vi "slide.vi"() -> ()   [LabVIEW 2023]
panel:
  in  "Tab Control":enum32{"Num Ctris", "Num Ctris i32"}(tab)
  in  "Knob":dbl(knob) scale=0.0..10.0
  in  "Dial":dbl(knob) scale=0.0..10.0
  in  "Vertical full Slide":dbl(slide) scale=0.0..10.0
  in  "Vertical Pointer Slide":dbl(slide) scale=0.0..10.0
  in  "Color Box":u32(colorbox)
  in  "Side Pointer Slide":dbl(slide) scale=0.0..10.0
  in  "Side Full Slide":dbl(slide) scale=0.0..10.0
  in  "Num Ctrl":dbl
  out "Numeric":dbl
  out "Side Full":dbl
  out "Side Pointer":dbl
  out "Vertical Full":dbl
  out "Vertical Pointer":dbl
  out "Knob_Value":dbl
  out "Dial Value":dbl
  out "Color DEC":u32
  out "Color BIN":u32 format="%b"
  out "Color OCT":u32 format="%o"
  out "Color HEX":u32 format="%x"
  in  "Knob 2":i32(knob) scale=0.0..10.0
  in  "Dial 2":i32(knob) scale=0.0..10.0
  in  "Vertical full Slide 2":i32(slide) scale=0.0..10.0
  in  "Vertical Pointer Slide  2":i32(slide) scale=0.0..10.0
  in  "Color Box 2":u32(colorbox)
  in  "Side Pointer Slide  2":i32(slide) scale=0.0..10.0
  in  "Side Full Slide  2":i32(slide) scale=0.0..10.0
  in  "Num Ctrl 2":i32
  out "Numeric 2":i32
  out "Side Full 2":i32
  out "Side Pointer 2":i32
  out "Vertical Full 2":i32
  out "Vertical Pointer 2":i32
  out "Knob_Value 2":i32
  out "Dial Value 2":i32
  out "u32 DEC":u32
  out "u32 HEX":u32 format="%x"
  out "u32 OCT":u32 format="%o"
  out "u32 BIN":u32 format="%b"
  in  "stop":bool
  # "Express内のNum  Ctrlsのアイコンの動きを知るためのVIです。\nDBL（少数を含む）とi32（整数）２種類の型で動きが確認できます。\nプログラム終了したい場合STOPボタンを押してください"
  # "型の変更方法"
  # "数字の表示設定方法"
  # "１．Representationを選択\n２．型を選択"
  # "１．Propertiesを選択\n２．Display Formatタグをクリック\n３．Typeを選択\n　Decimal：１０進数\n　Hexadecimal：１６進数\n　Octal：８進数\n　Binary：２進数"
  # "※Properties　Data Typeタグからも\n変更できます。"
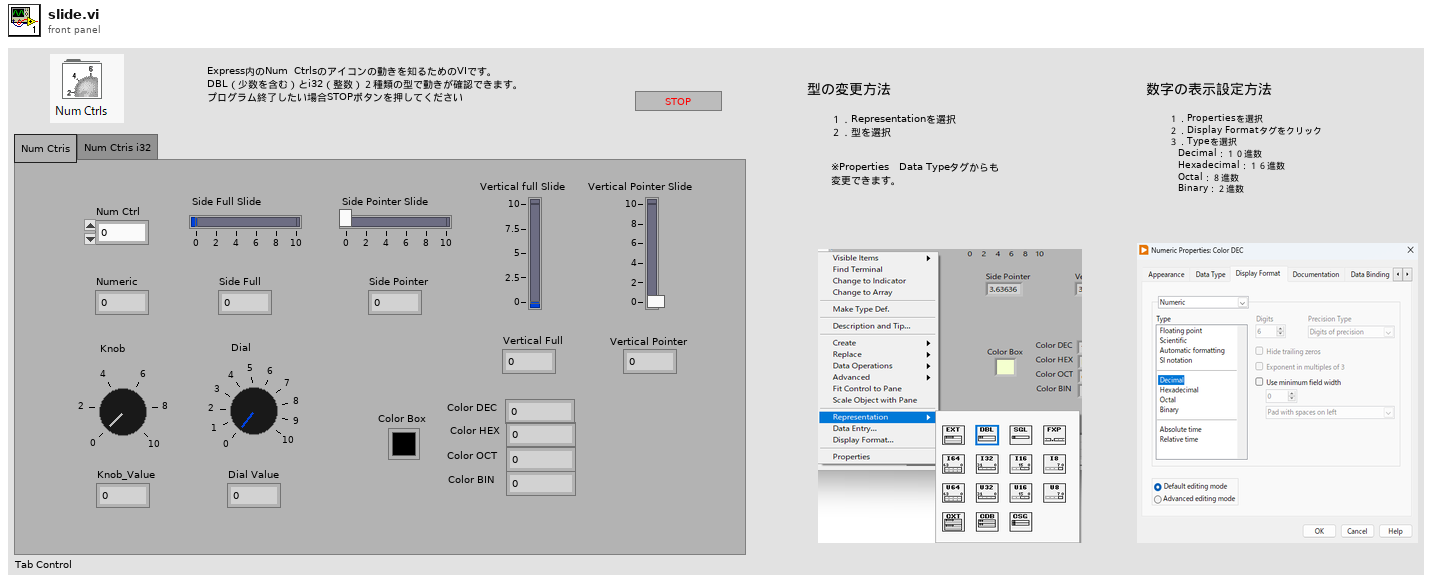
[diagram p1: front panel]
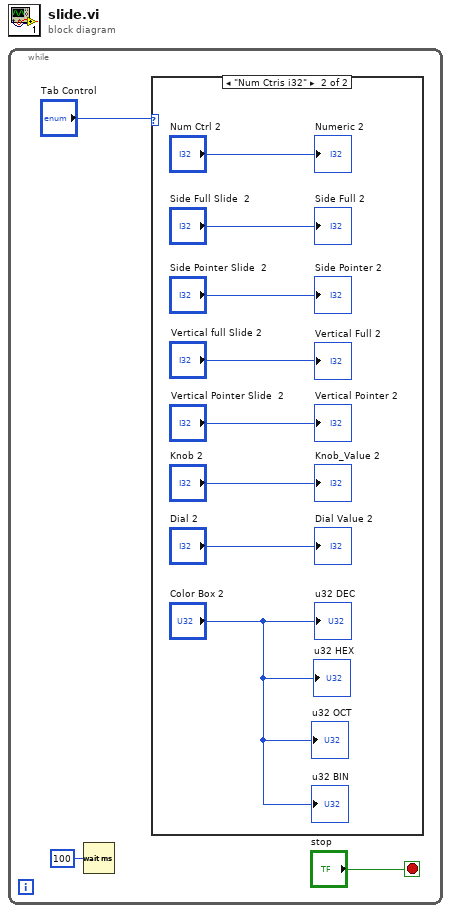
[diagram p0: block diagram]
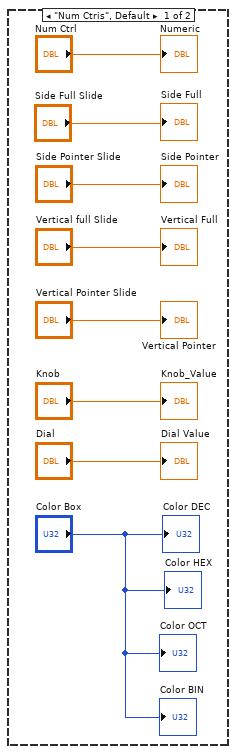
[diagram p2: hidden frame]
diagram:
  n1 = while {
    stop <- "stop" stop-if-true
    n2 = Wait (ms)(milliseconds to wait=u32 100) -> ()  [unwired: 1 out]
    n3 = case shown="\"Num Ctris i32\"" "Tab Control" {
      frame "Num Ctris", Default {
        "Vertical Pointer" <- "Vertical Pointer Slide"
        "Vertical Full" <- "Vertical full Slide"
        "Side Full" <- "Side Full Slide"
        "Side Pointer" <- "Side Pointer Slide"
        "Numeric" <- "Num Ctrl"
        "Knob_Value" <- "Knob"
        "Dial Value" <- "Dial"
        "Color DEC" <- "Color Box"
        "Color OCT" <- "Color Box"
        "Color BIN" <- "Color Box"
        "Color HEX" <- "Color Box"
      }
      frame "Num Ctris i32" {
        "u32 DEC" <- "Color Box 2"
        "Side Full 2" <- "Side Full Slide  2"
        "Knob_Value 2" <- "Knob 2"
        "Numeric 2" <- "Num Ctrl 2"
        "Vertical Full 2" <- "Vertical full Slide 2"
        "Dial Value 2" <- "Dial 2"
        "Side Pointer 2" <- "Side Pointer Slide  2"
        "Vertical Pointer 2" <- "Vertical Pointer Slide  2"
        "u32 HEX" <- "Color Box 2"
        "u32 OCT" <- "Color Box 2"
        "u32 BIN" <- "Color Box 2"
      }
    }
  }
